vi "Handle Error status bytes.vi"(8 "error in (no error)":errorcluster, 10 "Data in":u8[](array[numeric]) format="%x", 11 "Hist cluster":T1) -> (0 "error out":errorcluster)   [LabVIEW 2016]
uses:
  Typedefs/All ROBs info cluster refnum.ctl
  <vilib>/Utility/miscctls.llb/LVRowAndColumnTypeDef.ctl
  Global Variables/AllowUserMessages.vi
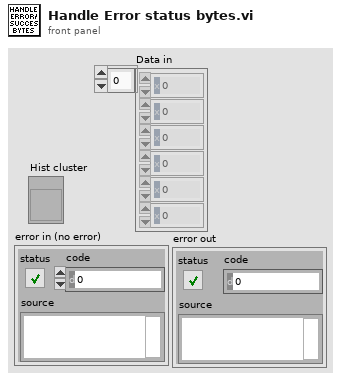
[diagram p1: front panel]
types:
  T1 = typedef "All ROBs info cluster refnum.ctl" = refnum<vi>
  T2 = cluster{"Long":i32, "Float":dbl, "Bool":bool, "Byte":u8, "Byte array":u8[]}
  T3 = enum16{"Byte array", "Byte", "Bool", "Long", "Float"}
  T4 = typedef "ROB info refnum.ctl" = refnum<vi>
  T5 = enum16{"ID", "Status", "Voltages", "Temp", "Latch count", "VRef", "Trigthres", "MPPC EN?", "Test charge?", "Responding?"}
  T6 = typedef "LVRowAndColumnTypeDef.ctl" = cluster{"Row":i32, "Column":i32}
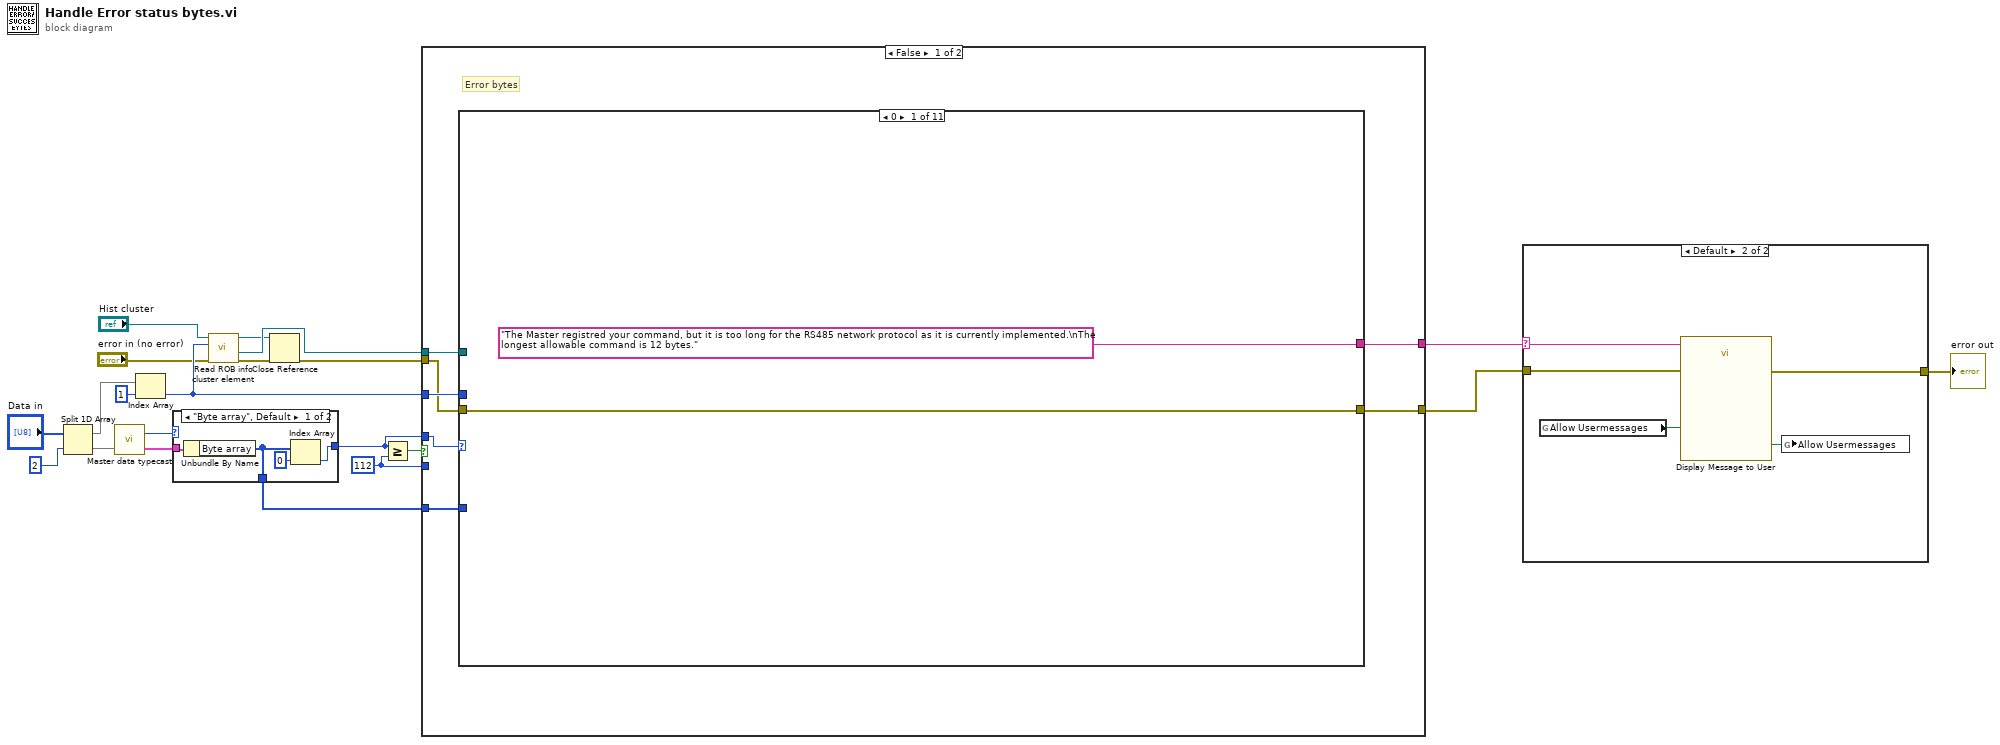
[diagram p0: block diagram]
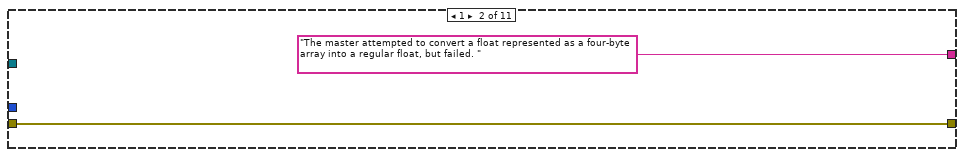
[diagram p3: hidden frame]
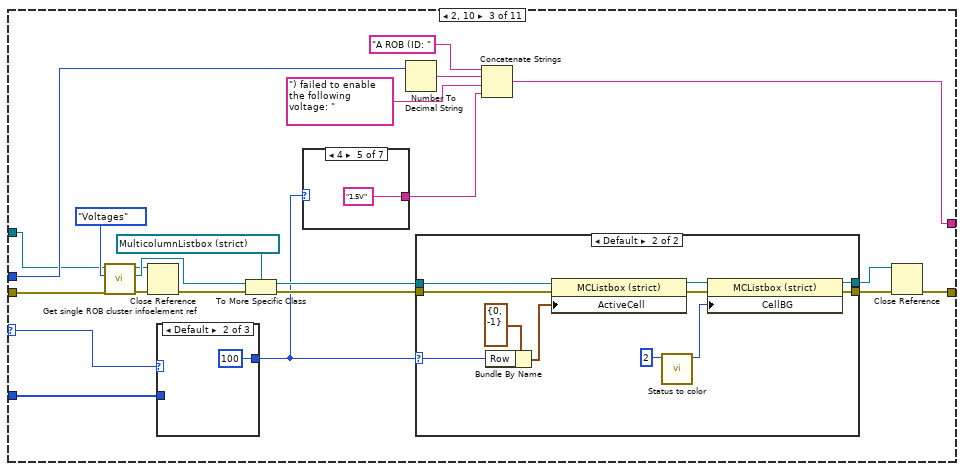
[diagram p4: hidden frame]
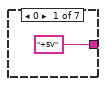
[diagram p6: hidden frame]
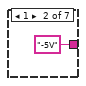
[diagram p7: hidden frame]
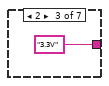
[diagram p8: hidden frame]
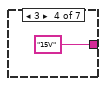
[diagram p9: hidden frame]
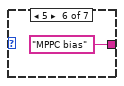
[diagram p10: hidden frame]
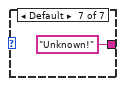
[diagram p11: hidden frame]
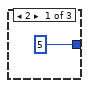
[diagram p12: hidden frame]
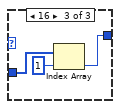
[diagram p13: hidden frame]
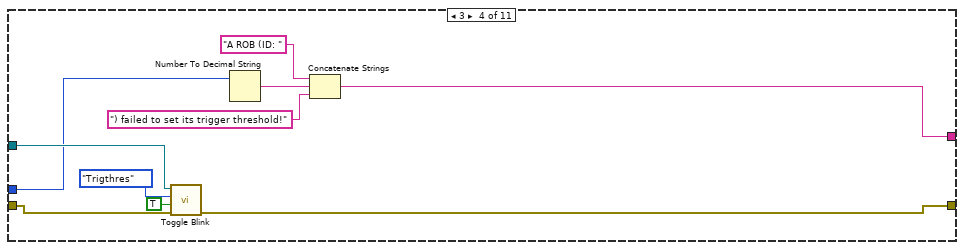
[diagram p14: hidden frame]
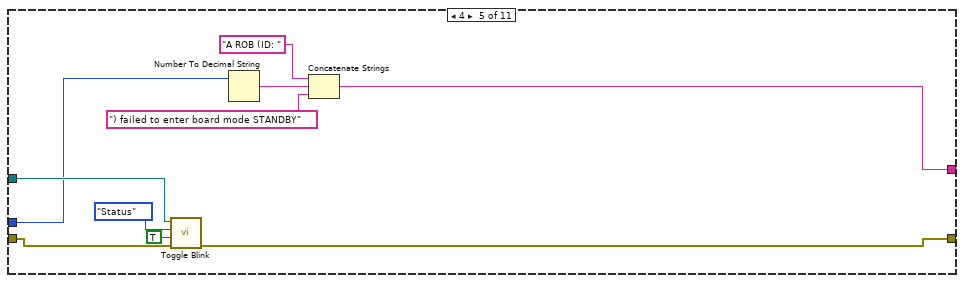
[diagram p15: hidden frame]
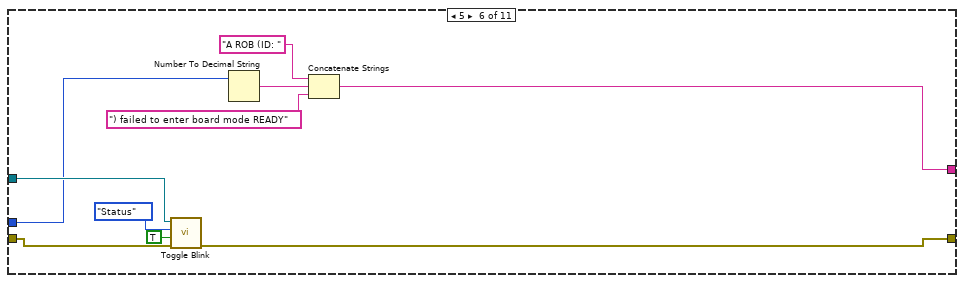
[diagram p16: hidden frame]
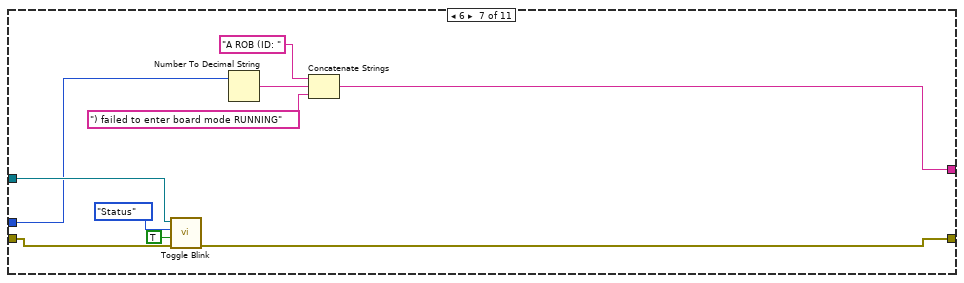
[diagram p17: hidden frame]
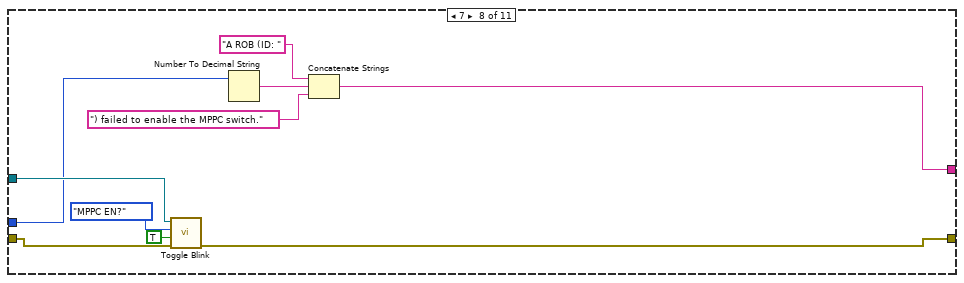
[diagram p18: hidden frame]
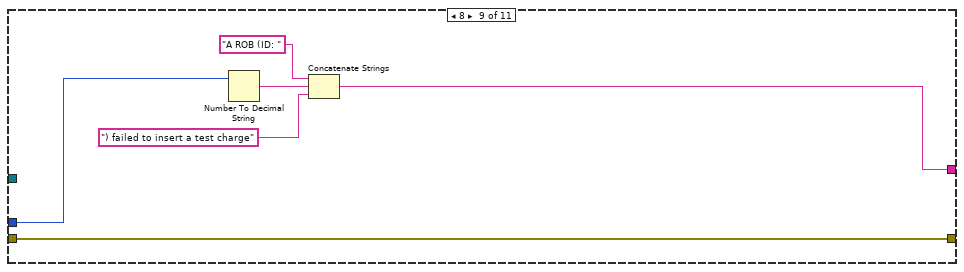
[diagram p19: hidden frame]
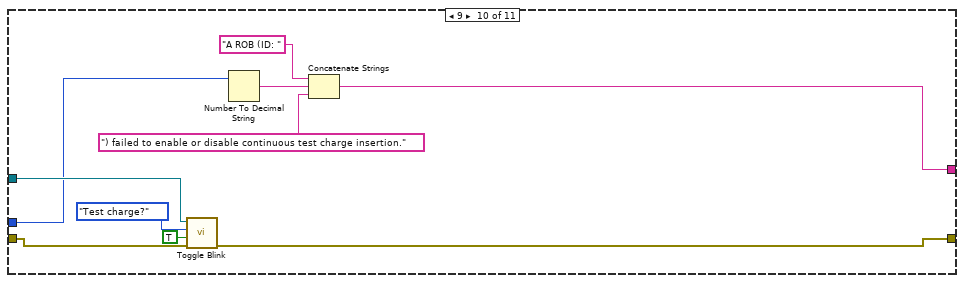
[diagram p20: hidden frame]
diagram:
  w5 = u8 112 ("Byte")
  n1 = Split 1D Array(array="Data in", index=2) -> (first subarray=w3:u8[], second subarray=w16:u8[])
  n2 = call "Master data typecast.vi"("Data in"=w16) -> ("Data out"=w18:T2, "Datatype"=w19:T3)  [unwired: 1 in]
  n3 = Index Array(array=w3, index=1) -> (element=w13:u8)
  n4 = case shown="\"Byte array\", Default" w19 {
    tunnel: w18 -> [w25 w27]
    tunnel: [w23 w26] -> w6
    tunnel: [w22 _] -> w15
    frame "Byte array", Default {
      n5 = Unbundle By Name(w25) -> ("Byte array"=w22:u8[])
      n6 = Index Array(array=w22, index=0) -> (element=w23:u8)
    }
    frame "Byte" {
      n7 = Unbundle By Name(w27) -> ("Byte"=w26:u8)
    }
  }
  n8 = call "Read ROB info cluster element.vi"("error in (no error)"="error in (no error)", "Channel"=w13, "ROB info clusters"="Hist cluster") -> ("error out"=w10:errorcluster, "ROB infocluster ref"=w11:T4, "ROB info clusters"=w9:T1)  [unwired: 5 in, 1 out]
  n9 = Close Reference(reference=w9, error in (no error)=w10) -> (error out=w8:errorcluster)
  n10 = Greater Or Equal?(x=w6, y=w5) -> (x >= y?=w7:bool)
  n11 = case shown="False" w7 {
    tunnel: w15 -> [w34 w158]
    tunnel: w13 -> [w33 w161]
    tunnel: w11 -> [w32 w160]
    tunnel: w8 -> [w31 w159]
    tunnel: [w30 w163] -> w1
    tunnel: [w29 w157] -> w4
    tunnel: w6 -> [w28 w165]
    tunnel: w5 -> [_ w164]
    frame False {
      # "Error bytes"
      n12 = case shown="0" w28 {
        selector: w28 -> [_ _ w55 _ _ _ _ _ _ _ w156]
        tunnel: ["The Master registred your command, but it is too long for the RS485 network protocol as it is currently implemented.\nThe longest allowable command is 12 bytes." "The master attempted to convert a float represented as a four-byte array into a regular float, but failed. " w48 w88 w98 w108 w118 w128 w137 w144 w153] -> w29
        tunnel: w33 -> [_ _ w53 w92 w102 w112 w122 w132 w141 w148 _]
        tunnel: w34 -> [_ _ w54 _ _ _ _ _ _ _ _]
        tunnel: w31 -> [w35 w37 w44 w93 w103 w113 w123 w133 w136 w149 w152]
        tunnel: w32 -> [_ _ w45 w94 w104 w114 w124 w134 _ w150 _]
        tunnel: [w35 w37 w40 w87 w97 w107 w117 w127 w136 w143 w152] -> w30
        frame 0 {
        }
        frame 1 {
        }
        frame 2, 10 {
          n13 = call "Get single ROB cluster infoelement ref.vi"("error in (no error)"=w44, "Enum"=T5."Voltages", "ROB infocluster ref"=w45) -> ("error out"=w43:errorcluster, "Element reference"=w59:refnum<vi>, "ROB infocluster ref"=w41:T4)  [unwired: 6 in]
          n14 = Close Reference(reference=w41, error in (no error)=w43) -> (error out=w42:errorcluster)
          n15 = case shown="Default" w55 {
            tunnel: [5 100 w83] -> w39
            tunnel: w54 -> [_ _ w85]
            frame 2 {
            }
            frame Default {
            }
            frame 16 {
              n16 = Index Array(array=w85, index=1) -> (element=w83:u8)
            }
          }
          n17 = To More Specific Class(target class=refnum<vi> refnum ("Voltages"), reference=w59, error in=w42) -> (specific class reference=w57:refnum<vi>, error out=w56:errorcluster)
          n18 = case shown="4" w39 {
            tunnel: ["+5V" "-5V" "3.3V" "15V" "1.5V" "MPPC bias" "Unknown!"] -> w49
            frame 0 {
            }
            frame 1 {
            }
            frame 2 {
            }
            frame 3 {
            }
            frame 4 {
            }
            frame 5 {
            }
            frame Default {
            }
          }
          n19 = Number To Decimal String(number=w53) -> (decimal integer string=w51:string)  [unwired: 1 in]
          n20 = case shown="Default" w39 {
            selector: w39 -> [_ w63]
            tunnel: w57 -> [w61 w73]
            tunnel: w56 -> [w62 w72]
            tunnel: [w62 w71] -> w47
            tunnel: [w61 w70] -> w46
            frame 100 {
            }
            frame Default {
              n21 = Bundle By Name(cluster=T6 {"Row"=0, "Column"=-1} ("Active Cell:Active Cell"), "Row"=w63) -> (w68:T6)
              n22 = property class="MCListbox (strict)"(reference=w73, error in=w72, "ActiveCell"=w68) -> (reference out=w67:refnum<vi>, error out=w66:errorcluster)
              n23 = call "Status to color.vi"("Byte"=u8 2) -> ("Numeric"=w65:u32)  [unwired: 10 in]
              n24 = property class="MCListbox (strict)"(reference=w67, error in=w66, "CellBG"=w65) -> (reference out=w70:refnum<vi>, error out=w71:errorcluster)
            }
          }
          n25 = Concatenate Strings("A ROB (ID: ", w51, ") failed to enable the following voltage: ", w49) -> (w48:string)
          n26 = Close Reference(reference=w46, error in (no error)=w47) -> (error out=w40:errorcluster)
        }
        frame 3 {
          n27 = call "Toggle Blink.vi"("error in (no error)"=w93, "Blinking"=TRUE, "Enum"=T5."Trigthres", "ROB infocluster ref"=w94) -> ("error out"=w87:errorcluster)  [unwired: 6 in, 1 out]
          n28 = Number To Decimal String(number=w92) -> (decimal integer string=w90:string)  [unwired: 1 in]
          n29 = Concatenate Strings("A ROB (ID: ", w90, ") failed to set its trigger threshold!") -> (w88:string)
        }
        frame 4 {
          n30 = call "Toggle Blink.vi"("error in (no error)"=w103, "Blinking"=TRUE, "Enum"=T5."Status", "ROB infocluster ref"=w104) -> ("error out"=w97:errorcluster)  [unwired: 6 in, 1 out]
          n31 = Number To Decimal String(number=w102) -> (decimal integer string=w100:string)  [unwired: 1 in]
          n32 = Concatenate Strings("A ROB (ID: ", w100, ") failed to enter board mode STANDBY") -> (w98:string)
        }
        frame 5 {
          n33 = call "Toggle Blink.vi"("error in (no error)"=w113, "Blinking"=TRUE, "Enum"=T5."Status", "ROB infocluster ref"=w114) -> ("error out"=w107:errorcluster)  [unwired: 6 in, 1 out]
          n34 = Number To Decimal String(number=w112) -> (decimal integer string=w110:string)  [unwired: 1 in]
          n35 = Concatenate Strings("A ROB (ID: ", w110, ") failed to enter board mode READY") -> (w108:string)
        }
        frame 6 {
          n36 = call "Toggle Blink.vi"("error in (no error)"=w123, "Blinking"=TRUE, "Enum"=T5."Status", "ROB infocluster ref"=w124) -> ("error out"=w117:errorcluster)  [unwired: 6 in, 1 out]
          n37 = Number To Decimal String(number=w122) -> (decimal integer string=w120:string)  [unwired: 1 in]
          n38 = Concatenate Strings("A ROB (ID: ", w120, ") failed to enter board mode RUNNING") -> (w118:string)
        }
        frame 7 {
          n39 = call "Toggle Blink.vi"("error in (no error)"=w133, "Blinking"=TRUE, "Enum"=T5."MPPC EN?", "ROB infocluster ref"=w134) -> ("error out"=w127:errorcluster)  [unwired: 6 in, 1 out]
          n40 = Number To Decimal String(number=w132) -> (decimal integer string=w130:string)  [unwired: 1 in]
          n41 = Concatenate Strings("A ROB (ID: ", w130, ") failed to enable the MPPC switch.") -> (w128:string)
        }
        frame 8 {
          n42 = Number To Decimal String(number=w141) -> (decimal integer string=w139:string)  [unwired: 1 in]
          n43 = Concatenate Strings("A ROB (ID: ", w139, ") failed to insert a test charge") -> (w137:string)
        }
        frame 9 {
          n44 = call "Toggle Blink.vi"("error in (no error)"=w149, "Blinking"=TRUE, "Enum"=T5."Test charge?", "ROB infocluster ref"=w150) -> ("error out"=w143:errorcluster)  [unwired: 6 in, 1 out]
          n45 = Number To Decimal String(number=w148) -> (decimal integer string=w146:string)  [unwired: 1 in]
          n46 = Concatenate Strings("A ROB (ID: ", w146, ") failed to enable or disable continuous test charge insertion.") -> (w144:string)
        }
        frame Default {
          n47 = Number To Hexadecimal String(2:w156) -> (0:w155:string)  [unwired: 1 in]
          n48 = Concatenate Strings("An error message was received from the master, but the error byte was not recognized.\nError byte: ", w155) -> (w153:string)
        }
      }
    }
    frame True {
      # "Success bytes"
      n49 = Subtract(x=w165, y=w164) -> (x-y=w162:u8)
      n50 = case shown="6" w162 {
        selector: w162 -> [_ w177 _ _ _ _ _ _ _ w235]
        tunnel: w161 -> [_ _ _ _ _ _ _ _ _ _]
        tunnel: w158 -> [_ w176 _ _ _ _ _ _ _ _]
        tunnel: w159 -> [w166 w172 w202 w207 w212 w217 w222 w225 w228 w232]
        tunnel: w160 -> [_ w173 w203 w208 w213 w218 w223 _ w229 _]
        tunnel: [w166 w168 w201 w206 w211 w216 w221 w225 w227 w232] -> w163
        tunnel: [_ _ _ _ _ _ _ _ _ w231] -> w157
        frame 0, 1 {
        }
        frame 2, 10 {
          n51 = call "Get single ROB cluster infoelement ref.vi"("error in (no error)"=w172, "Enum"=T5."Voltages", "ROB infocluster ref"=w173) -> ("error out"=w171:errorcluster, "Element reference"=w181:refnum<vi>, "ROB infocluster ref"=w169:T4)  [unwired: 6 in]
          n52 = Close Reference(reference=w169, error in (no error)=w171) -> (error out=w170:errorcluster)
          n53 = case shown="Default" w177 {
            tunnel: [5 100 w197] -> w167
            tunnel: w176 -> [_ _ w199]
            frame 2 {
            }
            frame Default {
            }
            frame 16 {
              n54 = Index Array(array=w199, index=1) -> (element=w197:u8)
            }
          }
          n55 = To More Specific Class(target class=refnum<vi> refnum ("Voltages"), reference=w181, error in=w170) -> (specific class reference=w179:refnum<vi>, error out=w178:errorcluster)
          n56 = case shown="Default" w167 {
            selector: w167 -> [_ w186]
            tunnel: w179 -> [w183 w194]
            tunnel: w178 -> [w184 w193]
            tunnel: [w184 w192] -> w175
            tunnel: [w183 w191] -> w174
            frame 100 {
            }
            frame Default {
              n57 = Bundle By Name(cluster=T6 {"Row"=0, "Column"=-1} ("Active Cell:Active Cell"), "Row"=w186) -> (w189:T6)
              n58 = property class="MCListbox (strict)"(reference=w194, error in=w193, "ActiveCell"=w189) -> (reference out=w188:refnum<vi>, error out=w187:errorcluster)
              n59 = property class="MCListbox (strict)"(reference=w188, error in=w187, "CellBG"=u32 11776947) -> (reference out=w191:refnum<vi>, error out=w192:errorcluster)
            }
          }
          n60 = Close Reference(reference=w174, error in (no error)=w175) -> (error out=w168:errorcluster)
        }
        frame 3 {
          n61 = call "Toggle Blink.vi"("error in (no error)"=w202, "Blinking"=FALSE, "Enum"=T5."Trigthres", "ROB infocluster ref"=w203) -> ("error out"=w201:errorcluster)  [unwired: 6 in, 1 out]
        }
        frame 4 {
          n62 = call "Toggle Blink.vi"("error in (no error)"=w207, "Blinking"=FALSE, "Enum"=T5."Status", "ROB infocluster ref"=w208) -> ("error out"=w206:errorcluster)  [unwired: 6 in, 1 out]
        }
        frame 5 {
          n63 = call "Toggle Blink.vi"("error in (no error)"=w212, "Blinking"=FALSE, "Enum"=T5."Status", "ROB infocluster ref"=w213) -> ("error out"=w211:errorcluster)  [unwired: 6 in, 1 out]
        }
        frame 6 {
          n64 = call "Toggle Blink.vi"("error in (no error)"=w217, "Blinking"=FALSE, "Enum"=T5."Status", "ROB infocluster ref"=w218) -> ("error out"=w216:errorcluster)  [unwired: 6 in, 1 out]
        }
        frame 7 {
          n65 = call "Toggle Blink.vi"("error in (no error)"=w222, "Blinking"=FALSE, "Enum"=T5."MPPC EN?", "ROB infocluster ref"=w223) -> ("error out"=w221:errorcluster)  [unwired: 6 in, 1 out]
        }
        frame 8 {
        }
        frame 9 {
          n66 = call "Toggle Blink.vi"("error in (no error)"=w228, "Blinking"=FALSE, "Enum"=T5."Test charge?", "ROB infocluster ref"=w229) -> ("error out"=w227:errorcluster)  [unwired: 6 in, 1 out]
        }
        frame Default {
          n67 = Number To Hexadecimal String(2:w235) -> (0:w234:string)  [unwired: 1 in]
          n68 = Concatenate Strings("An Success message was received from the master, but the error byte was not recognized.\nSuccess byte: ", w234) -> (w231:string)
        }
      }
    }
  }
  n69 = case shown="Default" w4 {
    selector: w4 -> [_ w241]
    tunnel: [w236 w238] -> w2
    tunnel: w1 -> [w236 w237]
    frame "" {
    }
    frame Default {
      n70 = global read "AllowUserMessages.vi" "Allow Usermessages"() -> (w239:bool)
      n71 = call "Display Message to User"("error in (no error)"=w237, "Enable"=w239, "Message"=w241) -> ("error out"=w238:errorcluster, "OK"=w240:bool)  [unwired: 7 in]
      n72 = global write "AllowUserMessages.vi" "Allow Usermessages"(w240) -> ()
    }
  }
  "error out" <- w2
